vi "Read StreamInfo.vi"(8 "error in (no error)":errorcluster, 11 "AODAcq in":refnum<class "AODAcq.lvclass">) -> (0 "error out":errorcluster, 2 "StreamInfo":T1, 3 "AODAcq out":refnum<class "AODAcq.lvclass">)   [LabVIEW 2011, in "AODAcq.lvclass"]
uses:
  AODAcq.lvclass
  AODAcq.lvclass/AODAcq.ctl
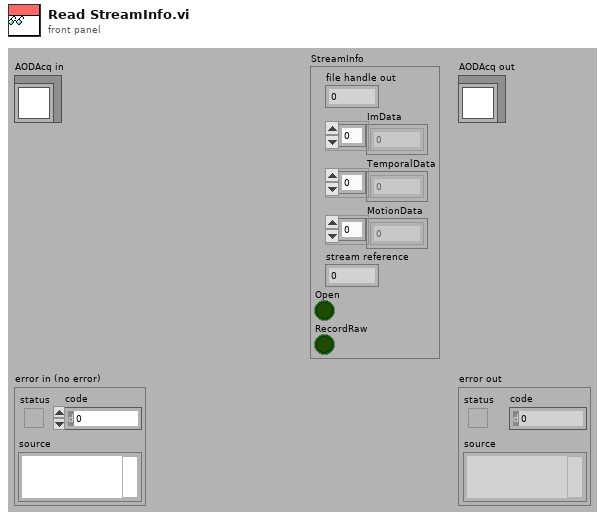
[diagram p1: front panel]
types:
  T1 = cluster{"file handle out":u32, "ImData":u32[], "TemporalData":u32[], "MotionData":u32[], "stream reference":u32, "Open":bool, "RecordRaw":bool}
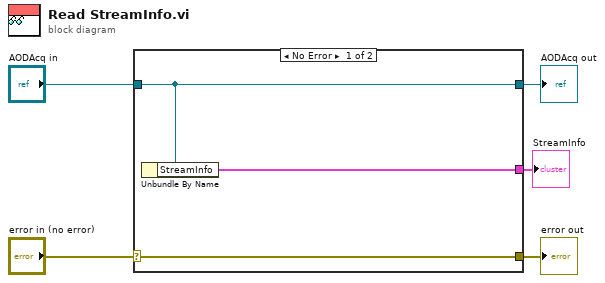
[diagram p0: block diagram]
diagram:
  n1 = case shown="No Error" "error in (no error)" {
    selector: "error in (no error)" -> [w8 w9]
    tunnel: [w8 w9] -> w4
    tunnel: [w7 w10] -> w2
    tunnel: "AODAcq in" -> [w7 w10]
    tunnel: [w6 _] -> w1
    frame No Error {
      n2 = Unbundle By Name(w7) -> ("StreamInfo"=w6:T1)
    }
    frame Error {
    }
  }
  "error out" <- w4
  "AODAcq out" <- w2
  "StreamInfo" <- w1
